vi "Create Camera Info.vi"(8 "FoV Y":dbl, 9 "FoV X":dbl, 10 "Y Image Resolution":i32, 11 "X Image Resolution":i32) -> (3 "Camera Info":T1)   [LabVIEW 2012]
uses:
  CameraResolutionInfo.ctl
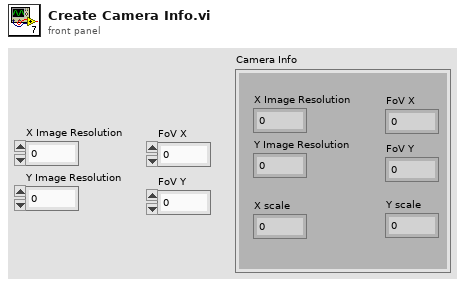
[diagram p1: front panel]
types:
  T1 = typedef "CameraResolutionInfo.ctl" = cluster{"X Image Resolution":i32, "Y Image Resolution":i32, "FoV X":dbl, "FoV Y":dbl, "X scale":dbl, "Y scale":dbl}
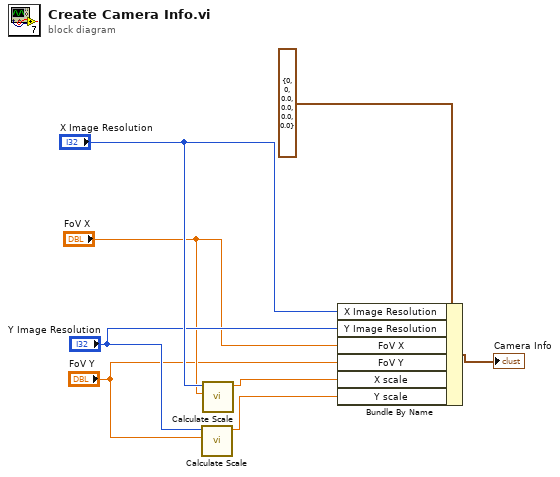
[diagram p0: block diagram]
diagram:
  n1 = call "Calculate Scale.vi"("FoV"="FoV Y", "Image Resolution"="Y Image Resolution") -> ("Scale"=w1:dbl)  [unwired: 9 in]
  n2 = call "Calculate Scale.vi"("FoV"="FoV X", "Image Resolution"="X Image Resolution") -> ("Scale"=w2:dbl)  [unwired: 9 in]
  n3 = Bundle By Name(cluster=T1 {"X Image Resolution"=0, "Y Image Resolution"=0, "FoV X"=0.0, "FoV Y"=0.0, "X scale"=0.0, "Y scale"=0.0} ("Camera Info 2"), "X Image Resolution"="X Image Resolution", "Y Image Resolution"="Y Image Resolution", "FoV X"="FoV X", "FoV Y"="FoV Y", "X scale"=w2, "Y scale"=w1) -> (→"Camera Info":T1)
